vi "UpdatePositionValue.vi"(5 "NewPositionValue":i32, 9 "Position in":T1, 10 "Device":string) -> (1 "UpdatedPosition":T1, 2 "DeviceOut":string)   [LabVIEW 2020, in "Picomotor8742.lvclass"]
uses:
  Picomotor8742.lvclass
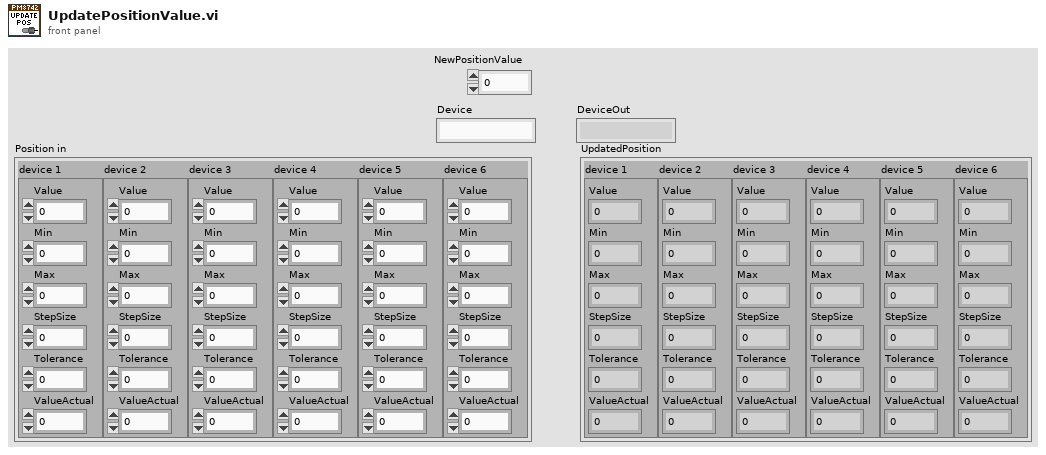
[diagram p1: front panel]
types:
  T1 = cluster{"device 1":cluster{"Value":dbl, "Min":dbl, "Max":dbl, "StepSize":dbl, "Tolerance":dbl, "ValueActual":dbl}, "device 2":cluster{"Value":dbl, "Min":dbl, "Max":dbl, "StepSize":dbl, "Tolerance":dbl, "ValueActual":dbl}, "device 3":cluster{"Value":dbl, "Min":dbl, "Max":dbl, "StepSize":dbl, "Tolerance":dbl, "ValueActual":dbl}, "device 4":cluster{"Value":dbl, "Min":dbl, "Max":dbl, "StepSize":dbl, "Tolerance":dbl, "ValueActual":dbl}, "device 5":cluster{"Value":dbl, "Min":dbl, "Max":dbl, "StepSize":dbl, "Tolerance":dbl, "ValueActual":dbl}, "device 6":cluster{"Value":dbl, "Min":dbl, "Max":dbl, "StepSize":dbl, "Tolerance":dbl, "ValueActual":dbl}}
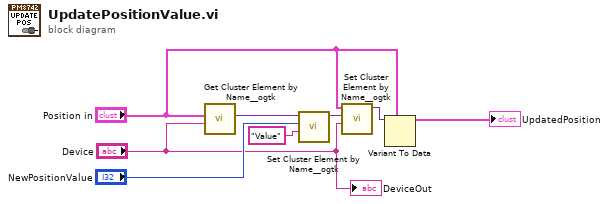
[diagram p0: block diagram]
diagram:
  n1 = call <userlib>:"Get Cluster Element by Name__ogtk.vi"("Element Name"="Device", "Cluster"="Position in") -> ("VElement"=w2:variant)  [unwired: 7 in, 2 out]
  n2 = call <userlib>:"Set Cluster Element by Name__ogtk.vi"("Element Name (\"\": New Element Data Name)"="Value" ("Element Name (\"\": New Element Data Name)"), "New Element Value"="NewPositionValue", "Cluster"=w2) -> ("VCluster out"=w4:variant)  [unwired: 6 in, 2 out]
  n3 = call <userlib>:"Set Cluster Element by Name__ogtk.vi"("Element Name (\"\": New Element Data Name)"="Device", "New Element Value"=w4, "Cluster"="Position in") -> ("VCluster out"=w5:variant)  [unwired: 6 in, 2 out]
  n4 = Variant To Data(type="Position in", Variant=w5) -> (data=→"UpdatedPosition":T1)  [unwired: 1 in, 1 out]
  "DeviceOut" <- "Device"
